vi "getDataPath.vi"(7 "LabVIEW Web Service Request":refnum<class "Web Request.lvclass">) -> ()   [LabVIEW 2016]
uses:
  <vilib>/wsapi/Web Request.lvclass
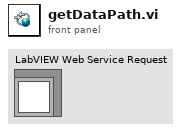
[diagram p1: front panel]
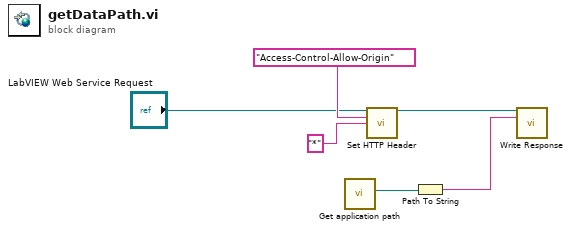
[diagram p0: block diagram]
diagram:
  n1 = call "Get application path.vi"() -> ("Application path"=w2:path)  [unwired: 11 in]
  n2 = call <vilib>:"Set HTTP Header.vi"("LabVIEW Web Service Request"="LabVIEW Web Service Request", "header"="Access-Control-Allow-Origin", "header value"="*") -> ("LabVIEW Web Service Request out"=w4:refnum<class "Web Request.lvclass">)  [unwired: 11 in, 1 out]
  n3 = Path To String(path=w2) -> (string=w1:string)
  n4 = call <vilib>:"Write Response.vi"("LabVIEW Web Service Request"=w4, "response string"=w1) -> ()  [unwired: 12 in, 2 out]
